vi "Tosca-Process DI.vi"(0 "Digital Inputs in":T1[](array[typedef]), 5 "Interval (ms)":dbl, 11 "DI":bool[](array[boolean])) -> (4 "Digital Inputs out":T1[](array[typedef]), 15 "DI out":bool[](array[boolean]))   [LabVIEW 2020]
uses:
  Tosca-Digital Input.ctl
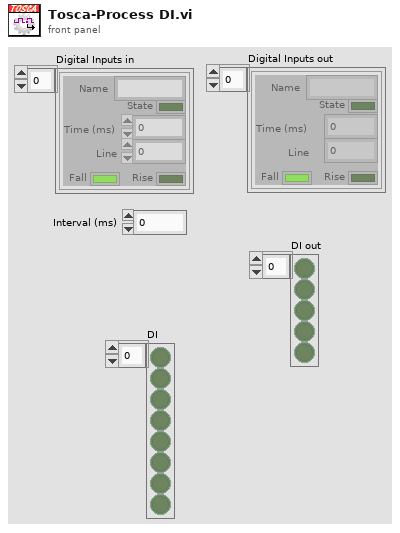
[diagram p1: front panel]
types:
  T1 = typedef "Tosca-Digital Input.ctl" = cluster{"Name":string, "State":bool, "Time (ms)":dbl, "Line":i32, "Rise":bool, "Fall":bool}
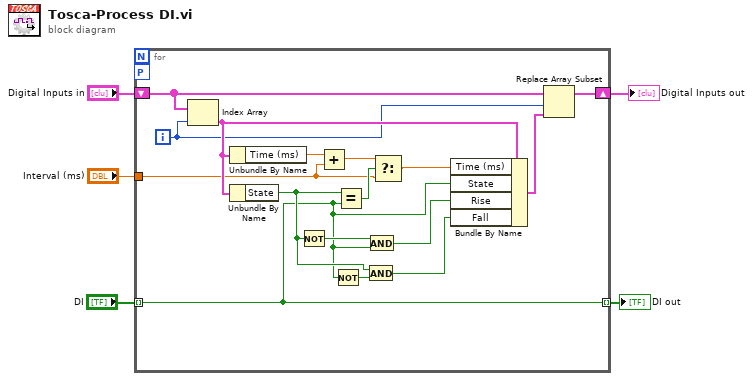
[diagram p0: block diagram]
diagram:
  n1 = for {
    tunnel: "DI" -> [w6] mode=indexing
    shift-right: [w19] -> w3
    shift-left: "Digital Inputs in" -> [w21]
    tunnel: "Interval (ms)" -> [w15]
    tunnel: [w6] -> w1 mode=indexing
    workers-P: _ -> [_]
    i -> [w7]
    n2 = Index Array(array=w21, index=w7) -> (element=w17:T1)
    n3 = Unbundle By Name(w17) -> ("Time (ms)"=w14:dbl)
    n4 = Unbundle By Name(w17) -> ("State"=w9:bool)
    n5 = Not(x=w9) -> (.not. x?=w12:bool)
    n6 = Add(x=w14, y=w15) -> (x+y=w16:dbl)
    n7 = Not(x=w6) -> (.not. x?=w10:bool)
    n8 = Equal?(x=w9, y=w6) -> (x = y?=w18:bool)
    n9 = And(x=w9, y=w10) -> (x .and. y?=w8:bool)
    n10 = And(x=w12, y=w6) -> (x .and. y?=w11:bool)
    n11 = Select(t=w16, s=w18, f=w15) -> (s? t:f=w13:dbl)
    n12 = Bundle By Name(cluster=w17, "Time (ms)"=w13, "State"=w6, "Rise"=w11, "Fall"=w8) -> (w20:T1)
    n13 = Replace Array Subset(array=w21, new element=w20, index=w7) -> (w19:T1[])
  }
  "Digital Inputs out" <- w3
  "DI out" <- w1
